vi "UpdateVIPBVersion.vi"(8 "error in (no error)":errorcluster, 10 "Updated Package Version":T1, 11 "Path to VIPB File":path) -> (2 "output":string, 3 "return code":i32)   [LabVIEW 2019]
uses:
  <vilib>/JKI/VIPM API/command-line/support/Version Info Cluster_vipm_api.ctl
  <vilib>/JKI/VIPM API/VIPM API_vipm_api.lvlib
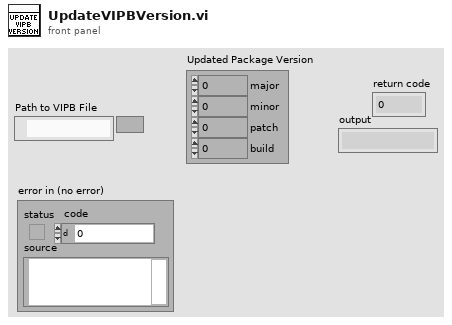
[diagram p1: front panel]
types:
  T1 = typedef "VIPM API_vipm_api.lvlib/Version Info Cluster_vipm_api.ctl" = cluster{"major":u32, "minor":u32, "patch":u32, "build":u32}
  T2 = typedef "VIPM API_vipm_api.lvlib/VI Package Build Spec Data Cluster_vipm_api.ctl" = cluster{"Package Version":T1, "Product Name":string, "Company Name":string, "Author Name (Person or Company)":string, "Product Homepage (URL)":string, "Legal Copyright":string, "License Agreement Name":string, "Product Description Summary":string, "Product Description":string, "Release Notes - Change Log":string}
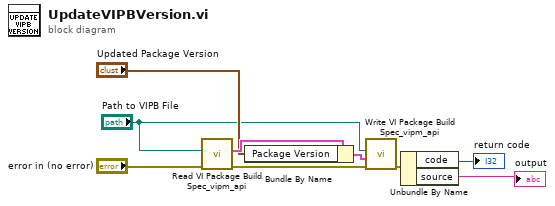
[diagram p0: block diagram]
diagram:
  n1 = call <vilib>:"Read VI Package Build Spec_vipm_api.vi"("error in (no error)"="error in (no error)", "Path to VIPB File"="Path to VIPB File") -> ("error out"=w6:errorcluster, "VI Package Build Spec Data"=w8:T2)  [unwired: 8 in]
  n2 = Bundle By Name(cluster=w8, "Package Version"="Updated Package Version") -> (w5:T2)
  n3 = call <vilib>:"Write VI Package Build Spec_vipm_api.vi"("error in (no error)"=w6, "VI Package Build Spec Data"=w5, "Path to VIPB File"="Path to VIPB File") -> ("error out"=w3:errorcluster)  [unwired: 8 in]
  n4 = Unbundle By Name(w3) -> ("code"=→"return code":i32, "source"=→"output":string)
